vi "Edge Detect.vi"(1 "Input":bool) -> (0 "Falling Edge":bool, 2 "RisingEdge":bool)   [LabVIEW 2012, in "ProcessorHelperFunctions.lvlib"]
uses:
  ProcessorHelperFunctions.lvlib
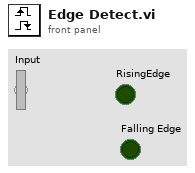
[diagram p1: front panel]
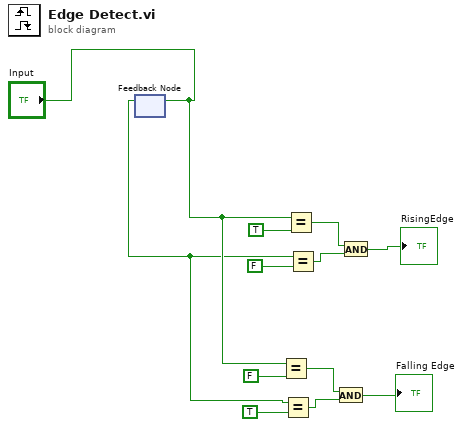
[diagram p0: block diagram]
diagram:
  n1 = feedback-in #1("Input") -> ()
  n2 = feedback #1() -> (w1:bool)  [unwired: 1 in]
  n3 = Equal?(x="Input", y=FALSE) -> (x = y?=w7:bool)
  n4 = Equal?(x=w1, y=TRUE) -> (x = y?=w6:bool)
  n5 = Equal?(x="Input", y=TRUE) -> (x = y?=w11:bool)
  n6 = Equal?(x=w1, y=FALSE) -> (x = y?=w10:bool)
  n7 = And(x=w7, y=w6) -> (x .and. y?=→"Falling Edge":bool)
  n8 = And(x=w11, y=w10) -> (x .and. y?=→"RisingEdge":bool)
